vi "Install Source.vi"() -> ()   [LabVIEW 2011, in "LVH-Build-Tools.lvlib"]
doc: "This VI will copy the source files into the install directory and create hard links replace the source files with hard links to the install directory.\n\nNote: Do not open any VI's from the source directory. All edits should be done in the Install directory to preserve paths."
uses:
  LVH-Build-Tools.lvlib
panel:
  out "Components":string[](array[string])
  out "Install Root":string
  out "Source Root":string
  out "Deleted From Souce":path[](array[path])
  # "Install Source"
  # "1. Run this VI\n2. When prompted select the config.ini file for the project you are working on.  The config.ini should be in the soure root directory.\n3. This VI will copy the source files into the install directory and create hard links replace the source files with hard links to the install directory.\n\nNote: Do not open any VI's from the source directory.  All edits should be done in the Install directory to preserve paths."
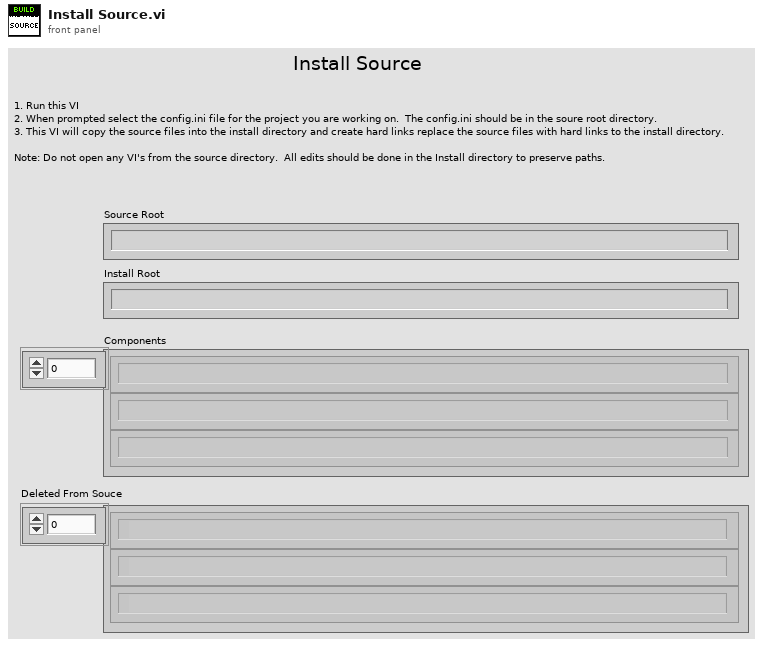
[diagram p1: front panel]
types:
  T1 = typedef "LVH-Build-Tools.lvlib/Configuration.ctl" = cluster{"Source Root":string, "Install Root":string, "Components":string[], "Ignore":string[]}
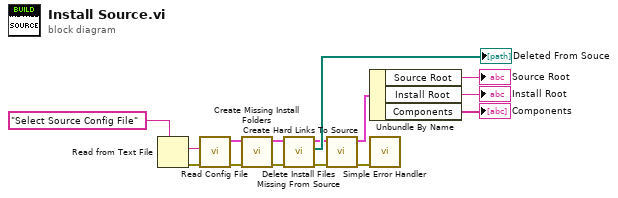
[diagram p0: block diagram]
diagram:
  n1 = Read from Text File(prompt (Open existing file)="Select Source Config File") -> (text=w13:string, error out=w15:errorcluster)  [unwired: 3 in, 2 out]
  n2 = call "Read Config File.vi"("error in (no error)"=w15, "Config File In"=w13) -> ("error out"=w11:errorcluster, "Configuration out"=w10:T1)  [unwired: 8 in]
  n3 = call "Create Missing Install Folders.vi"("Error In"=w11, "Configuration"=w10) -> ("Error Out"=w8:errorcluster, "Configuration"=w9:T1)  [unwired: 8 in]
  n4 = call "Delete Install Files Missing From Source.vi"("Error In"=w8, "Configuration"=w9) -> ("Error Out"=w6:errorcluster, "Deleted From Souce"=→"Deleted From Souce":path[], "Configuration"=w7:T1)  [unwired: 7 in]
  n5 = call "Create Hard Links To Source.vi"("Error In"=w6, "Configuration"=w7) -> ("Error Out"=w5:errorcluster, "Configuration"=w4:T1)  [unwired: 8 in]
  n6 = Unbundle By Name(w4) -> ("Source Root"=→"Source Root":string, "Install Root"=→"Install Root":string, "Components"=→"Components":string[])
  n7 = call <vilib>:"Simple Error Handler.vi"("error in (no error)"=w5) -> ()  [unwired: 4 in, 5 out]
